vi "Close SP.vi"(8 "error in (no error)":errorcluster, 11 "Subpanel-Abstract in":refnum<class "Subpanel-Abstract.lvclass">) -> (0 "error out":errorcluster, 3 "Subpanel-Abstract out":refnum<class "Subpanel-Abstract.lvclass">)   [LabVIEW 2023, in "Data Analysis.lvlib" / "Subpanel-Abstract.lvclass"]
uses:
  Subpanel-Abstract.lvclass
  Subpanel-Abstract.lvclass/Subpanel-Abstract.ctl
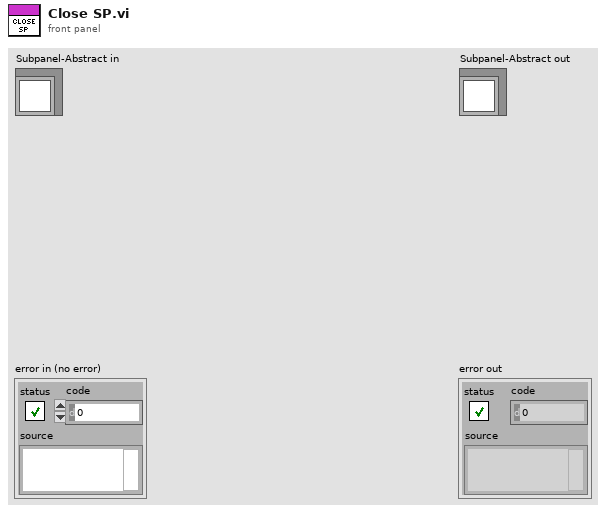
[diagram p1: front panel]
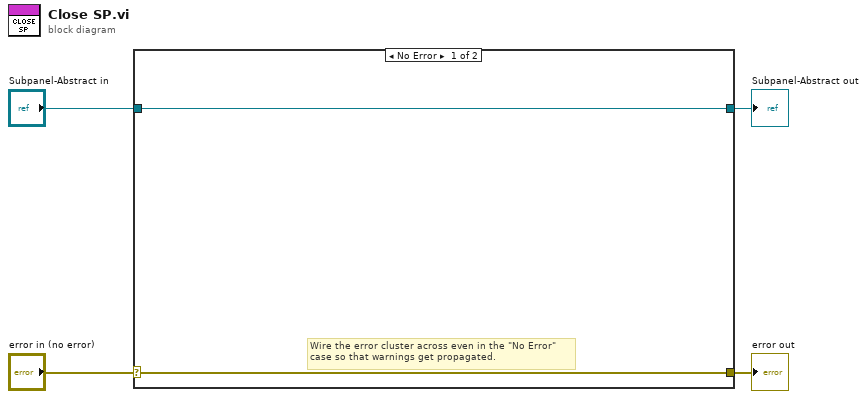
[diagram p0: block diagram]
diagram:
  n1 = case shown="No Error" "error in (no error)" {
    selector: "error in (no error)" -> [w6 w8]
    tunnel: [w6 w8] -> w3
    tunnel: [w5 w7] -> w1
    tunnel: "Subpanel-Abstract in" -> [w5 w7]
    frame No Error {
      # "Wire the error cluster across even in the \"No Error\"\ncase so that warnings get propagated."
    }
    frame Error {
    }
  }
  "error out" <- w3
  "Subpanel-Abstract out" <- w1
